vi "NI32LV110ASD4_Build DashBoard Data.vi"(11 "Dashboard Enables":T3={"Analog Module 1"=[TRUE, TRUE, TRUE, TRUE, TRUE, TRUE, TRUE, TRUE], "Analog Module 2"=[FALSE, FALSE, FALSE, FALSE, FALSE, FALSE, FALSE, FALSE], "Digital Module 1"=TRUE, "Digital Module 2"=FALSE, "Solenoid Module"=TRUE, "Turret Gyro"=FALSE, "Robot Gyro"=FALSE, "Left Encoder"=FALSE, "Launcher Rate"=FALSE, "Right Encoder"=FALSE}) -> ()   [LabVIEW 2011]
doc: "This VI builds data and sends it back to the dashboard PC program. By default it sends back the raw values for the first analog, digital, and solenoid module. Modify it to send back the data you want to view. Consider adding higher level data to the Dashboard Datatype.ctl and to this VI. Then update the Dashboard to display the data however you like.\n\nThis software is licensed. Open the labview\\readme\\WPI Robotics Library Open Source License.txt file for more information."
uses:
  Dashboard Datatype.ctl
  <vilib>/Rock Robotics/WPI/DriverStation/WPI_DriverStationDigitalData.ctl
panel:
  out "Dashboard Data":T1
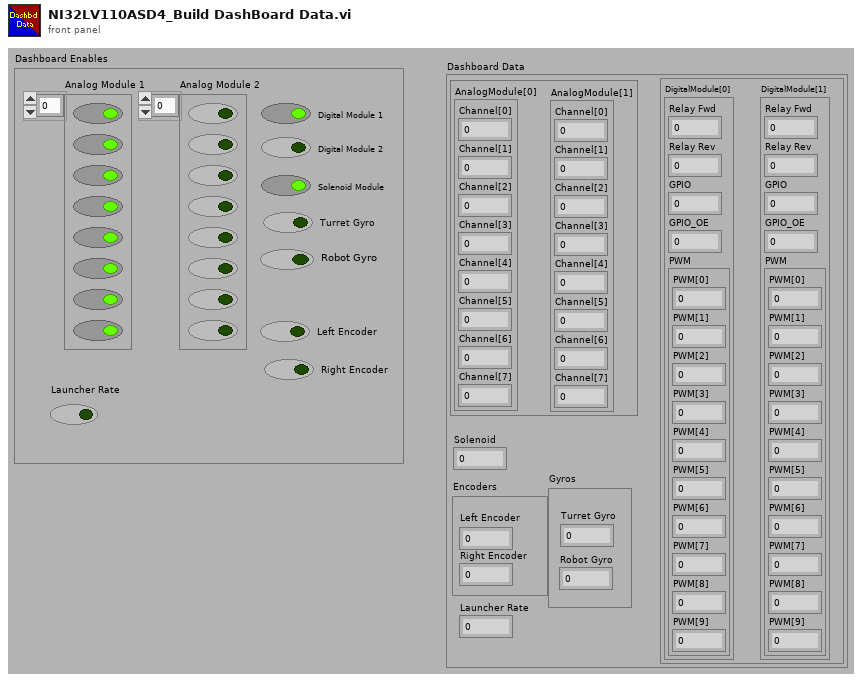
[diagram p1: front panel]
types:
  T1 = typedef "Dashboard Datatype.ctl" = cluster{cluster{"AnalogModule[0]":cluster{"Channel[0]":sgl, "Channel[1]":sgl, "Channel[2]":sgl, "Channel[3]":sgl, "Channel[4]":sgl, "Channel[5]":sgl, "Channel[6]":sgl, "Channel[7]":sgl}, "AnalogModule[1]":cluster{"Channel[0]":sgl, "Channel[1]":sgl, "Channel[2]":sgl, "Channel[3]":sgl, "Channel[4]":sgl, "Channel[5]":sgl, "Channel[6]":sgl, "Channel[7]":sgl}}, cluster{"DigitalModule[0]":T2, "DigitalModule[1]":T2}, "Solenoid":u8, "Launcher Rate":dbl, "Gyros":cluster{"Turret Gyro":dbl, "Robot Gyro":dbl}, "Encoders":cluster{"Left Encoder":dbl, "Right Encoder":dbl}}
  T2 = typedef "WPI_DriverStationDigitalData.ctl" = cluster{"Relay Fwd":u8, "Relay Rev":u8, "GPIO":u16, "GPIO_OE":u16, "PWM":cluster{"PWM[0]":u8, "PWM[1]":u8, "PWM[2]":u8, "PWM[3]":u8, "PWM[4]":u8, "PWM[5]":u8, "PWM[6]":u8, "PWM[7]":u8, "PWM[8]":u8, "PWM[9]":u8}}
  T3 = cluster{"Analog Module 1":bool[], "Analog Module 2":bool[], "Digital Module 1":bool, "Digital Module 2":bool, "Solenoid Module":bool, "Turret Gyro":bool, "Robot Gyro":bool, "Left Encoder":bool, "Launcher Rate":bool, "Right Encoder":bool}
  T4 = cluster{"AnalogModule[0]":cluster{"Channel[0]":sgl, "Channel[1]":sgl, "Channel[2]":sgl, "Channel[3]":sgl, "Channel[4]":sgl, "Channel[5]":sgl, "Channel[6]":sgl, "Channel[7]":sgl}, "AnalogModule[1]":cluster{"Channel[0]":sgl, "Channel[1]":sgl, "Channel[2]":sgl, "Channel[3]":sgl, "Channel[4]":sgl, "Channel[5]":sgl, "Channel[6]":sgl, "Channel[7]":sgl}}
  T5 = cluster{"Channel[0]":sgl, "Channel[1]":sgl, "Channel[2]":sgl, "Channel[3]":sgl, "Channel[4]":sgl, "Channel[5]":sgl, "Channel[6]":sgl, "Channel[7]":sgl}[]
  T6 = cluster{"Channel[0]":sgl, "Channel[1]":sgl, "Channel[2]":sgl, "Channel[3]":sgl, "Channel[4]":sgl, "Channel[5]":sgl, "Channel[6]":sgl, "Channel[7]":sgl}
  T7 = cluster{"AnalogModule[0][0]":sgl, "AnalogModule[0][1]":sgl, "AnalogModule[0][2]":sgl, "AnalogModule[0][3]":sgl, "AnalogModule[0][4]":sgl, "AnalogModule[0][5]":sgl, "AnalogModule[0][6]":sgl, "AnalogModule[0][7]":sgl}
  T8 = cluster{"[0]":cluster{"Channel[0]":sgl, "Channel[1]":sgl, "Channel[2]":sgl, "Channel[3]":sgl, "Channel[4]":sgl, "Channel[5]":sgl, "Channel[6]":sgl, "Channel[7]":sgl}, "[1]":cluster{"Channel[0]":sgl, "Channel[1]":sgl, "Channel[2]":sgl, "Channel[3]":sgl, "Channel[4]":sgl, "Channel[5]":sgl, "Channel[6]":sgl, "Channel[7]":sgl}}
  T9 = cluster{"DigitalModule[0]":T2, "DigitalModule[1]":T2}
  T10 = typedef "FPGA_DIODevRef.ctl" = cluster{"DevStatus":errorcluster, "Module":T11}
  T11 = typedef "FPGA_TypedefDigitalModule.ctl" = enum16{"Digital Module 1", "Digital Module 2"}
  T12 = cluster{"[0]":u8, "[1]":u8, "[2]":u8, "[3]":u8, "[4]":u8, "[5]":u8, "[6]":u8, "[7]":u8, "[8]":u8, "[9]":u8}
  T13 = typedef "FPGA_SolenoidDevRef.ctl" = cluster{"DevStatus":errorcluster, "Module":T14}
  T14 = typedef "FPGA_TypedefSolenoidModule.ctl" = enum16{"Solenoid Module 1", "Solenoid Module 2"}
  T15 = typedef "WPI_EncoderDevRef.ctl" = cluster{"DevStatus":errorcluster, "EncoderIndex":T16, "CounterIndex":T17, "DistancePerCount":dbl, "Decoding Type":T18}
  T16 = typedef "FPGA_EncoderIdx.ctl" = enum8{"Enc 0", "Enc 1", "Enc 2", "Enc 3", "Invalid"}
  T17 = typedef "FPGA_CounterCtrSystemIndex.ctl" = enum8{"Ctr 0", "Ctr 1", "Ctr 2", "Ctr 3", "Ctr 4", "Ctr 5", "Ctr 6", "Ctr 7", "Invalid"}
  T18 = typedef "WPI_EncoderType.ctl" = enum16{"1x", "2x", "4x"}
  T19 = typedef "WPI_GyroDevRef.ctl" = cluster{"DevStatus":errorcluster, "Analog Module":T20, "Analog Channel":T21, "Offset":dbl, "Gain (VoltsPerDegree/Second)":dbl}
  T20 = typedef "FPGA_TypedefAnalogModule.ctl" = enum16{"Analog Module 1", "Analog Module 2"}
  T21 = typedef "FPGA_AIChannel.ctl" = enum8{"AI 1", "AI 2", "AI 3", "AI 4", "AI 5", "AI 6", "AI 7", "AI 8", "Invalid"}
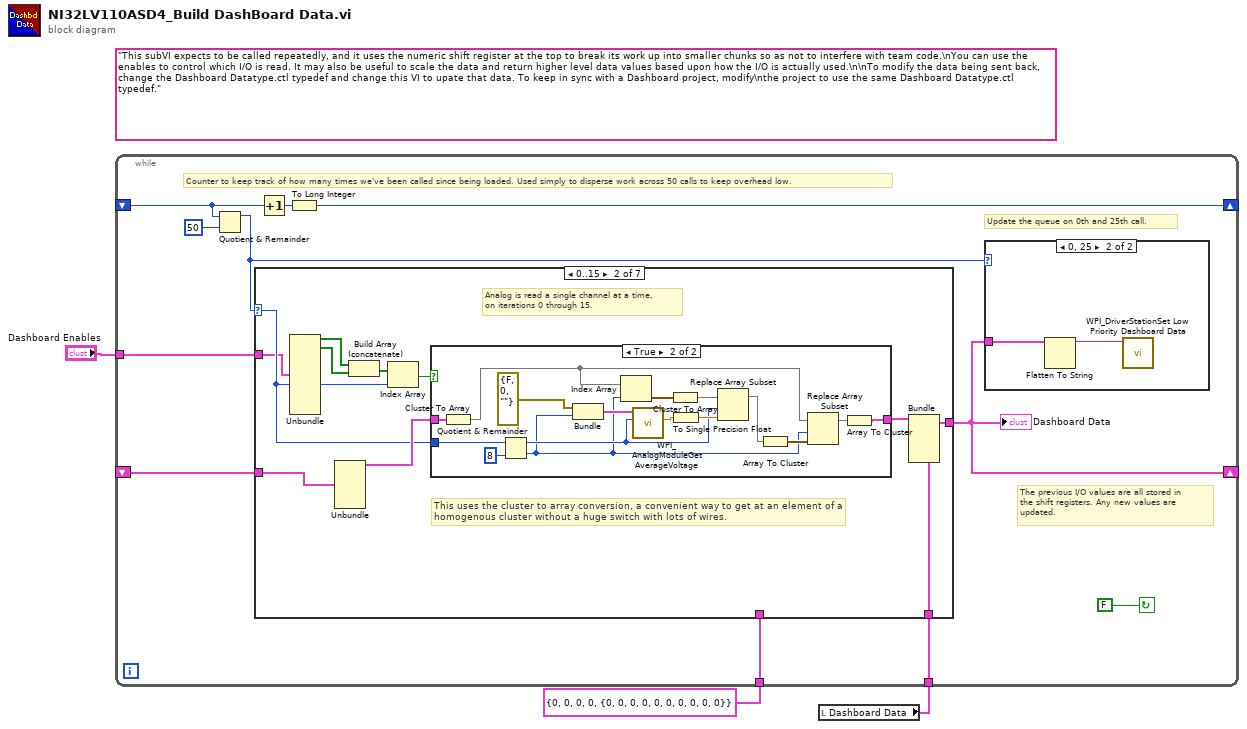
[diagram p0: block diagram]
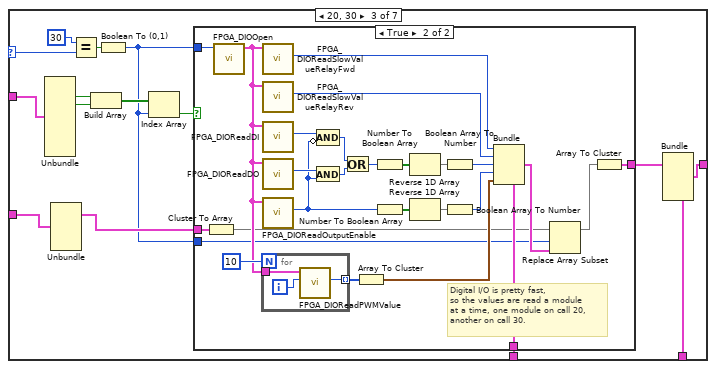
[diagram p5: hidden frame]
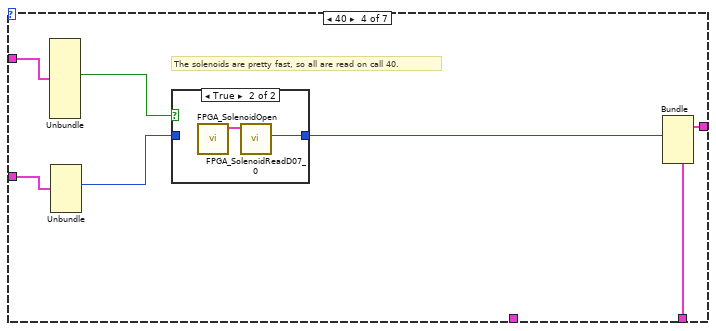
[diagram p7: hidden frame]
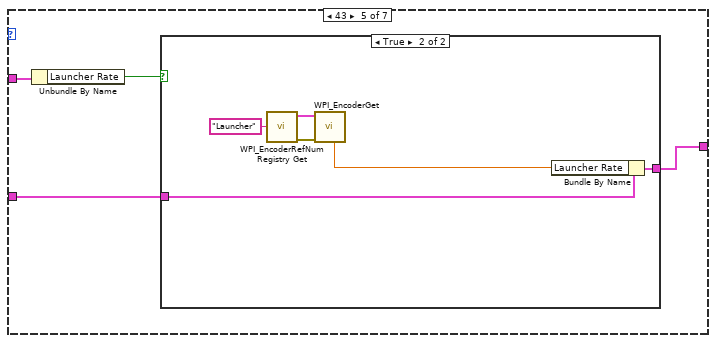
[diagram p9: hidden frame]
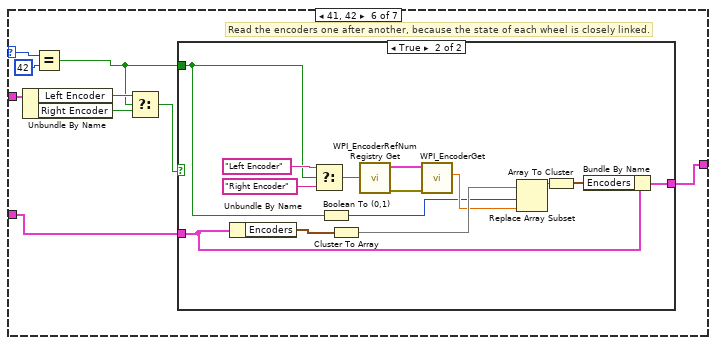
[diagram p11: hidden frame]
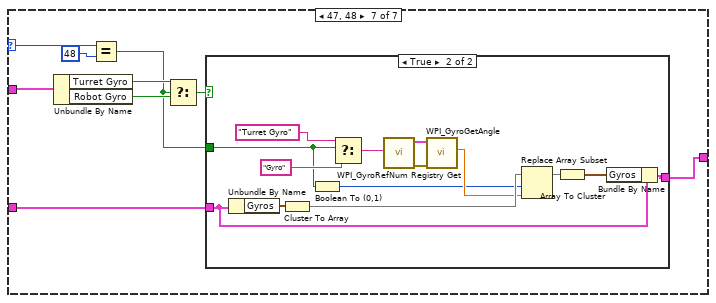
[diagram p13: hidden frame]
diagram:
  (unwired) "This subVI expects to be called repeatedly, and it uses the numeric shift register at the top to break its work up into smaller chunks so as not to interfere with team code.\nYou can use the enables to control which I/O is read. It may also be useful to scale the data and return higher level data values based upon how the I/O is actually used.\n\nTo modify the data being sent back, change the Dashboard Datatype.ctl typedef and change this VI to upate that data. To keep in sync with a Dashboard project, modify\nthe project to use the same Dashboard Datatype.ctl typedef."
  n1 = local read "Dashboard Data"() -> (w2:T1)
  n2 = while {
    shift-right: [w7] -> _
    shift-left: _ -> [w9]
    shift-right: [w4] -> _
    shift-left: _ -> [w12]
    tunnel: T2 {"Relay Fwd"=0, "Relay Rev"=0, "GPIO"=0, "GPIO_OE"=0, "PWM"={"PWM[0]"=0, "PWM[1]"=0, "PWM[2]"=0, "PWM[3]"=0, "PWM[4]"=0, "PWM[5]"=0, "PWM[6]"=0, "PWM[7]"=0, "PWM[8]"=0, "PWM[9]"=0}} ("DigitalModule[1]") -> [w11]
    tunnel: w2 -> [w6]
    tunnel: "Dashboard Enables" -> [w5]
    stop <- FALSE continue-if-true
    # "Counter to keep track of how many times we've been called since being loaded. Used simply to disperse work across 50 calls to keep overhead low."
    # "Update the queue on 0th and 25th call."
    # "The previous I/O values are all stored in\nthe shift registers. Any new values are\nupdated."
    n3 = Quotient & Remainder(x=w9, y=50) -> (x-y*floor(x/y)=w8:i32)  [unwired: 1 out]
    n4 = case shown="0..15" w8 {
      selector: w8 -> [_ w23 w56 _ _ w120 w141]
      tunnel: [w17 w19 w47 w94 w102 w112 w136] -> w4
      tunnel: w12 -> [w17 w18 w49 w96 w101 w113 w137]
      tunnel: w11 -> [_ _ w60 _ _ _ _]
      tunnel: w6 -> [_ w25 w48 w93 _ _ _]
      tunnel: w5 -> [_ w22 w54 w97 w104 w118 w144]
      frame Default {
        # "Don't update any I/O"
      }
      frame 0..15 {
        # "This uses the cluster to array conversion, a convenient way to get at an element of a\nhomogenous cluster without a huge switch with lots of wires."
        # "Analog is read a single channel at a time,\non iterations 0 through 15."
        n5 = Unbundle(w22) -> ("Analog Module 1"=w21:bool[], "Analog Module 2"=w20:bool[])  [unwired: 8 out]
        n6 = Unbundle(w18) -> (w24:T4)  [unwired: 5 out]
        n7 = Build Array (concatenate)(w21, w20) -> (w27:bool[])
        n8 = Index Array(array=w27, index=w23) -> (element=w28:bool)
        n9 = case shown="True" w28 {
          tunnel: w23 -> [_ w36]
          tunnel: [w29 w33] -> w26
          tunnel: w24 -> [w29 w32]
          frame False {
          }
          frame True {
            n10 = Cluster To Array(cluster=w32) -> (array=w30:T5)
            n11 = Quotient & Remainder(x=w36, y=8) -> (x-y*floor(x/y)=w35:i32, floor(x/y)=w31:i32)
            n12 = Bundle("DevStatus"=errorcluster {"status"=FALSE, "code"=0, "source"=""}, w31) -> (w44:cluster{"DevStatus":errorcluster, i32})  [unwired: 1 out]
            n13 = Index Array(array=w30, index=w31) -> (element=w38:T6)
            n14 = call <vilib>:"WPI_AnalogModuleGetAverageVoltage.vi"("Channel"=w35, "AnalogModuleDevStatus"=w44) -> ("Average Voltage"=w41:dbl)  [unwired: 1 in, 8 out]
            n15 = Cluster To Array(cluster=w38) -> (array=w37:sgl[])
            n16 = To Single Precision Float(number=w41) -> (single precision float=w40:sgl)
            n17 = Replace Array Subset(array=w37, new element=w40, index=w35) -> (w39:sgl[])
            n18 = Array To Cluster(array=w39) -> (cluster=w43:T7)
            n19 = Replace Array Subset(array=w30, new element=w43, index=w31) -> (w34:T5)
            n20 = Array To Cluster(array=w34) -> (cluster=w33:T8)
          }
        }
        n21 = Bundle(cluster=w25, w26) -> (w19:T1)  [unwired: 5 out]
      }
      frame 20, 30 {
        n22 = Unbundle(w54) -> ("Digital Module 1"=w53:bool, "Digital Module 2"=w52:bool)  [unwired: 8 out]
        n23 = Unbundle(w49) -> (w51:T9)  [unwired: 5 out]
        n24 = Equal?(x=30, y=w56) -> (x = y?=w58:bool)
        n25 = Build Array(w53, w52) -> (w55:bool[])
        n26 = Boolean To (0,1)(Boolean=w58) -> (0, 1=w46:i16)
        n27 = Index Array(array=w55, index=w46) -> (element=w57:bool)
        n28 = case shown="True" w57 {
          tunnel: w60 -> [_ w69]
          tunnel: [w61 w62] -> w50
          tunnel: w46 -> [_ w67]
          tunnel: w46 -> [_ w66]
          tunnel: w51 -> [w61 w65]
          frame False {
          }
          frame True {
            # "Digital I/O is pretty fast,\nso the values are read a module\nat a time, one module on call 20,\nanother on call 30."
            n29 = Cluster To Array(cluster=w65) -> (array=w64:T2[])
            n30 = call <vilib>:"FPGA_DIOOpen.vi"("Module (Module 1)"=w67) -> ("DIODeviceRef"=w85:T10)  [unwired: 1 in, 9 out]
            n31 = for {
              N: 10 -> [_]
              tunnel: w85 -> [w90]
              tunnel: [w88] -> w86 mode=indexing
              i -> [w89]
              n32 = call <vilib>:"FPGA_DIOReadPWMValue.vi"("PWMChannel"=w89, "DIODeviceRef In"=w90) -> ("PWMValue"=w88:u8)  [unwired: 1 in, 8 out]
            }
            n33 = call <vilib>:"FPGA_DIOReadSlowValueRelayFwd.vi"("DIODeviceRef In"=w85) -> ("Relay Forward"=w78:u8)  [unwired: 1 in, 9 out]
            n34 = call <vilib>:"FPGA_DIOReadSlowValueRelayRev.vi"("DIODeviceRef In"=w85) -> ("Relay Reverse"=w79:u8)  [unwired: 1 in, 9 out]
            n35 = call <vilib>:"FPGA_DIOReadDI.vi"("DIODeviceRef In"=w85) -> ("DI"=w83:u16)  [unwired: 1 in, 9 out]
            n36 = call <vilib>:"FPGA_DIOReadDO.vi"("DIODeviceRef In"=w85) -> ("DO"=w82:u16)  [unwired: 1 in, 9 out]
            n37 = call <vilib>:"FPGA_DIOReadOutputEnable.vi"("DIODeviceRef In"=w85) -> ("OutputEnable"=w73:u16)  [unwired: 1 in, 9 out]
            n38 = And(x=w82, y=w73) -> (x .and. y?=w81:u16)
            n39 = Compound Arithmetic op=AND(w83, invert w73) -> (w80:u16)
            n40 = Or(x=w80, y=w81) -> (x .or. y?=w71:u16)
            n41 = Array To Cluster(array=w86) -> (cluster=w84:T12)
            n42 = Number To Boolean Array(number=w71) -> (Boolean array=w76:bool[])
            n43 = Number To Boolean Array(number=w73) -> (Boolean array=w75:bool[])
            n44 = Reverse 1D Array(array=w76) -> (reversed array=w77:bool[])
            n45 = Reverse 1D Array(array=w75) -> (reversed array=w74:bool[])
            n46 = Boolean Array To Number(Boolean array=w77) -> (number=w70:u32)
            n47 = Boolean Array To Number(Boolean array=w74) -> (number=w72:u32)
            n48 = Bundle(cluster=w69, "Relay Fwd"=w78, "Relay Rev"=w79, "GPIO"=w70, "GPIO_OE"=w72, "PWM"=w84) -> (w68:T2)
            n49 = Replace Array Subset(array=w64, new element=w68, index=w66) -> (w63:T2[])
            n50 = Array To Cluster(array=w63) -> (cluster=w62:cluster{"[0]":T2, "[1]":T2})
          }
        }
        n51 = Bundle(cluster=w48, w50) -> (w47:T1)  [unwired: 5 out]
      }
      frame 40 {
        # "The solenoids are pretty fast, so all are read on call 40."
        n52 = Unbundle(w97) -> ("Solenoid Module"=w91:bool)  [unwired: 9 out]
        n53 = Unbundle(w96) -> ("Solenoid"=w95:u8)  [unwired: 5 out]
        n54 = case shown="True" w91 {
          tunnel: [w98 w99] -> w92
          tunnel: w95 -> [w98 _]
          frame False {
          }
          frame True {
            n55 = call <vilib>:"FPGA_SolenoidOpen.vi"() -> ("SolenoidDevRef"=w100:T13)  [unwired: 2 in, 9 out]
            n56 = call <vilib>:"FPGA_SolenoidReadD07_0.vi"("SolenoidDevRef"=w100) -> ("DO7:0"=w99:u8)  [unwired: 1 in, 9 out]
          }
        }
        n57 = Bundle(cluster=w93, "Solenoid"=w92) -> (w94:T1)  [unwired: 5 out]
      }
      frame 43 {
        n58 = Unbundle By Name(w104) -> ("Launcher Rate"=w103:bool)
        n59 = case shown="True" w103 {
          tunnel: [w105 w108] -> w102
          tunnel: w101 -> [w105 w107]
          frame False {
          }
          frame True {
            n60 = call <vilib>:"WPI_EncoderRefNum Registry Get.vi"("refnum name"="Launcher") -> ("error out"=w110:errorcluster, "EncoderDevRef"=w109:T15)  [unwired: 9 in]
            n61 = call <vilib>:"WPI_EncoderGet.vi"("error in (no error)"=w110, "EncoderDevRef"=w109) -> ("Rate"=w106:dbl)  [unwired: 4 in, 5 out]
            n62 = Bundle By Name(cluster=w107, "Launcher Rate"=w106) -> (w108:T1)
          }
        }
      }
      frame 41, 42 {
        # "Read the encoders one after another, because the state of each wheel is closely linked."
        n63 = Unbundle By Name(w118) -> ("Left Encoder"=w116:bool, "Right Encoder"=w117:bool)
        n64 = Equal?(x=w120, y=42) -> (x = y?=w115:bool)
        n65 = Select(t=w116, s=w115, f=w117) -> (s? t:f=w114:bool)
        n66 = case shown="True" w114 {
          tunnel: w115 -> [_ w127]
          tunnel: w113 -> [w121 w124]
          tunnel: [w121 w123] -> w112
          frame False {
          }
          frame True {
            n67 = Unbundle By Name(w124) -> ("Encoders"=w130:cluster{"Left Encoder":dbl, "Right Encoder":dbl})
            n68 = Select(t="Left Encoder" ("refnum name"), s=w127, f="Right Encoder") -> (s? t:f=w131:string)
            n69 = Boolean To (0,1)(Boolean=w127) -> (0, 1=w126:i16)
            n70 = Cluster To Array(cluster=w130) -> (array=w129:dbl[])
            n71 = call <vilib>:"WPI_EncoderRefNum Registry Get.vi"("refnum name"=w131) -> ("error out"=w134:errorcluster, "EncoderDevRef"=w135:T15)  [unwired: 9 in]
            n72 = call <vilib>:"WPI_EncoderGet.vi"("error in (no error)"=w134, "EncoderDevRef"=w135) -> ("Distance"=w128:dbl)  [unwired: 4 in, 5 out]
            n73 = Replace Array Subset(array=w129, new element=w128, index=w126) -> (w125:dbl[])
            n74 = Array To Cluster(array=w125) -> (cluster=w122:cluster{"Encoders[0]":dbl, "Encoders[1]":dbl})
            n75 = Bundle By Name(cluster=w124, "Encoders"=w122) -> (w123:T1)
          }
        }
      }
      frame 47, 48 {
        n76 = Unbundle By Name(w144) -> ("Turret Gyro"=w143:bool, "Robot Gyro"=w142:bool)
        n77 = Equal?(x=w141, y=48) -> (x = y?=w138:bool)
        n78 = Select(t=w143, s=w138, f=w142) -> (s? t:f=w139:bool)
        n79 = case shown="True" w139 {
          tunnel: w138 -> [_ w154]
          tunnel: w137 -> [w145 w148]
          tunnel: [w145 w150] -> w136
          frame False {
          }
          frame True {
            n80 = Unbundle By Name(w148) -> ("Gyros"=w147:cluster{"Turret Gyro":dbl, "Robot Gyro":dbl})
            n81 = Cluster To Array(cluster=w147) -> (array=w153:dbl[])
            n82 = Boolean To (0,1)(Boolean=w154) -> (0, 1=w149:i16)
            n83 = Select(t="Turret Gyro", s=w154, f="Gyro") -> (s? t:f=w155:string)
            n84 = call <vilib>:"WPI_GyroRefNum Registry Get.vi"("refnum name"=w155) -> ("error out"=w159:errorcluster, "GyroDevRef"=w158:T19)  [unwired: 9 in]
            n85 = call <vilib>:"WPI_GyroGetAngle.vi"("error in (no error)"=w159, "GyroDevRef"=w158) -> ("Angle"=w152:dbl)  [unwired: 6 in, 3 out]
            n86 = Replace Array Subset(array=w153, new element=w152, index=w149) -> (w151:dbl[])
            n87 = Array To Cluster(array=w151) -> (cluster=w146:cluster{"Gyros[0]":dbl, "Gyros[1]":dbl})
            n88 = Bundle By Name(cluster=w148, "Gyros"=w146) -> (w150:T1)
          }
        }
      }
    }
    "Dashboard Data" <- w4
    n89 = Increment(x=w9) -> (x+1=w14:i32)
    n90 = To Long Integer(number=w14) -> (32bit integer=w7:i32)
    n91 = case shown="0, 25" w8 {
      tunnel: w4 -> [_ w16]
      frame Default {
      }
      frame 0, 25 {
        n92 = Flatten To String(anything=w16) -> (data string=w15:string)  [unwired: 1 in, 4 out]
        n93 = call <vilib>:"WPI_DriverStationSet Low Priority Dashboard Data.vi"("User Data"=w15) -> ()  [unwired: 1 in, 10 out]
      }
    }
  }
